vi "test_Elements Remaining Channel Waveform Incoming.vi"(8 "error in (no error)":errorcluster, 11 "TestCase in":refnum<class "DMA Waveform Status Channel Testing.lvclass">) -> (0 "error out":errorcluster, 3 "TestCase out":refnum<class "DMA Waveform Status Channel Testing.lvclass">)   [LabVIEW 2019, in "DMA Waveform Status Channel Testing.lvclass"]
uses:
  DMA Waveform Status Channel Testing.lvclass
  <vilib>/addons/_JKI Toolkits/VI Tester/TestCase.llb/TestCase.lvclass
  C:/Program Files (x86)/National Instruments/LabVIEW 2019/vi.lib/addons/_JKI Toolkits/VI Tester/TestCase.llb/TestCase.lvclass
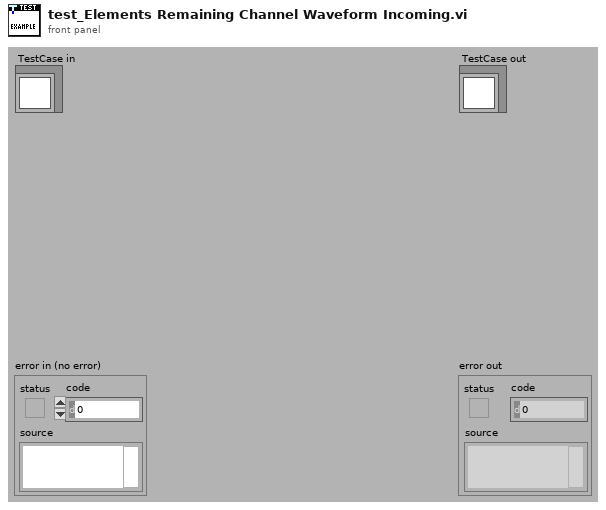
[diagram p1: front panel]
types:
  T1 = typedef "NI_VS Workspace ExecutionAPI.lvlib/WorkspaceAPI.ctl" = refnum<k24>
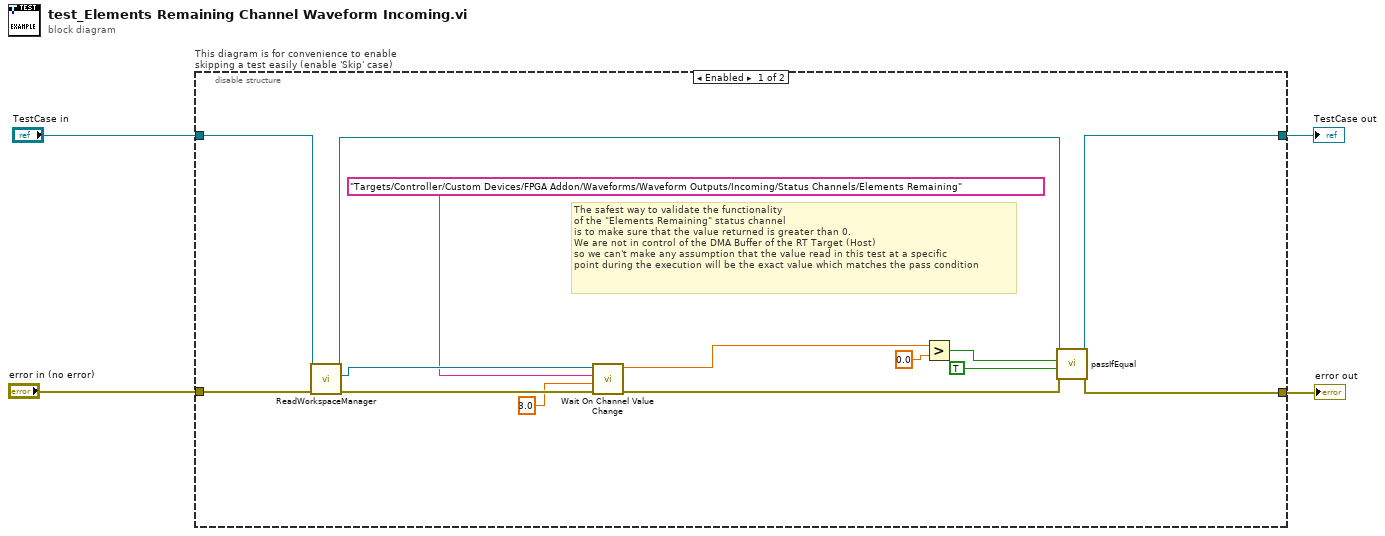
[diagram p0: block diagram]
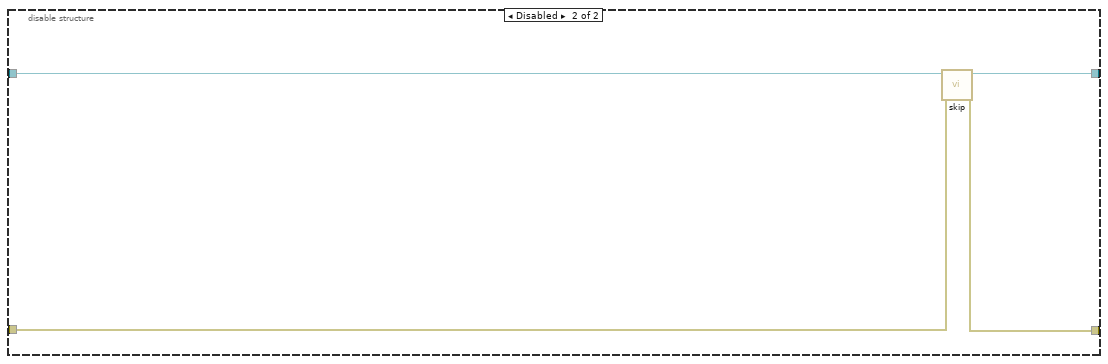
[diagram p2: hidden frame]
diagram:
  n1 = disable-structure "This diagram is for convenience to enable skipping a test easily (enable 'Skip' case)" shown="Enabled" {
    disable-tunnel: "TestCase in" -> [w12 w22]
    disable-tunnel: [w18 w20] -> w1
    disable-tunnel: [w17 w21] -> w3
    disable-tunnel: "error in (no error)" -> [w15 w19]
    frame Enabled {
      # "The safest way to validate the functionality\nof the \"Elements Remaining\" status channel\nis to make sure that the value returned is greater than 0.\nWe are not in control of the DMA Buffer of the RT Target (Host)\nso we can't make any assumption that the value read in this test at a specific \npoint during the execution will be the exact value which matches the pass condition"
      n2 = call-dynamic "ReadWorkspaceManager.vi"("error in (no error)"=w15, "VeriStand Test Case in"=w12) -> ("error out"=w16:errorcluster, "Workspace"=w14:T1, "VeriStand Test Case out"=w13:refnum<class "DMA Waveform Status Channel Testing.lvclass">)  [unwired: 7 in]
      n3 = call "Wait On Channel Value Change.vi"("error in (no error)"=w16, "Time to Wait"=3.0, "Channel"="Targets/Controller/Custom Devices/FPGA Addon/Waveforms/Waveform Outputs/Incoming/Status Channels/Elements Remaining", ".NET Refnum in"=w14) -> ("error out"=w11:errorcluster, "Value"=w8:dbl)  [unwired: 6 in]
      n4 = Greater?(x=w8, y=0.0) -> (0:w6:bool)
      n5 = call-dynamic "passIfEqual.vi"("error in (no error)"=w11, "y"=TRUE, "x"=w6, "TestCase in"=w13) -> ("error out"=w17:errorcluster, "TestCase out"=w18:refnum<class "DMA Waveform Status Channel Testing.lvclass">)  [unwired: 6 in]
    }
    frame Disabled {
      # "skip test result while test is under development"
      n6 = call <vilib>:"skip.vi"("error in (no error)"=w19, "TestCase in"=w22) -> ("error out"=w21:errorcluster, "TestCase out"=w20:refnum<class "DMA Waveform Status Channel Testing.lvclass">)  [unwired: 8 in]
    }
  }
  "error out" <- w3
  "TestCase out" <- w1
